vi "Persistent.vi"(7 "Field monitor ref":refnum<vi>, 8 "error in (no error)":errorcluster, 10 "Go to persistent mode?":bool, 11 "Power Supply in":refnum<class "Power Supply.lvclass">) -> (0 "error out":errorcluster, 3 "Power Supply out":refnum<class "Power Supply.lvclass">)   [LabVIEW 2009, in "Power Supply.lvclass"]
doc: "Persistent mode closes the switch and turns off the power supply. The superconducting electromagnet will then remain energized indefinitely.\n\nTo leave persistent mode, you must first ramp up the power supply to match the energized magnet, then open the switch. \n\nA current mismatch is dangerous! The magnet will forbid opening the switch unless the power supply matches the energized magnet."
uses:
  Power Supply.lvclass
  Global/Relative Sound Files.vi
panel:
  out "SHon?":bool caption="Switch Heater"
  out "persis?":bool caption="Persistent"
  out "title":string
  out "Field":dbl[unit]
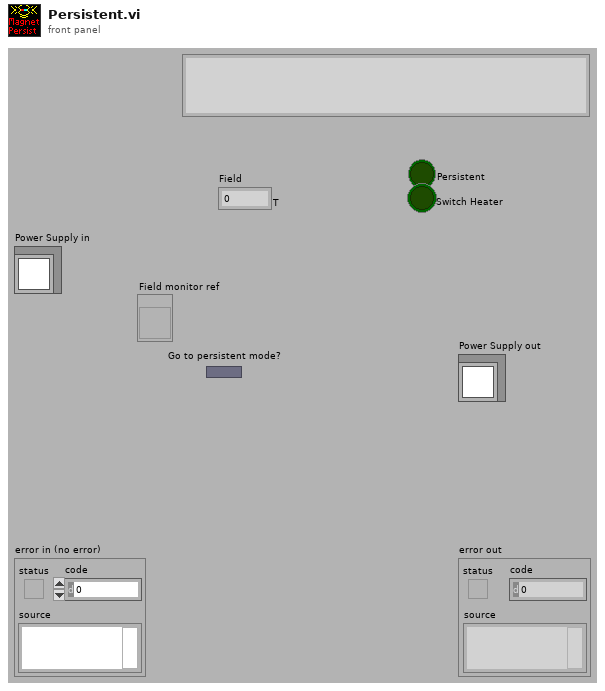
[diagram p1: front panel]
types:
  T1 = typedef "Power Supply.lvclass/Switch Heater Status.ctl" = enum16{"Off (at zero)", "On", "Off (at field)", "Other"}
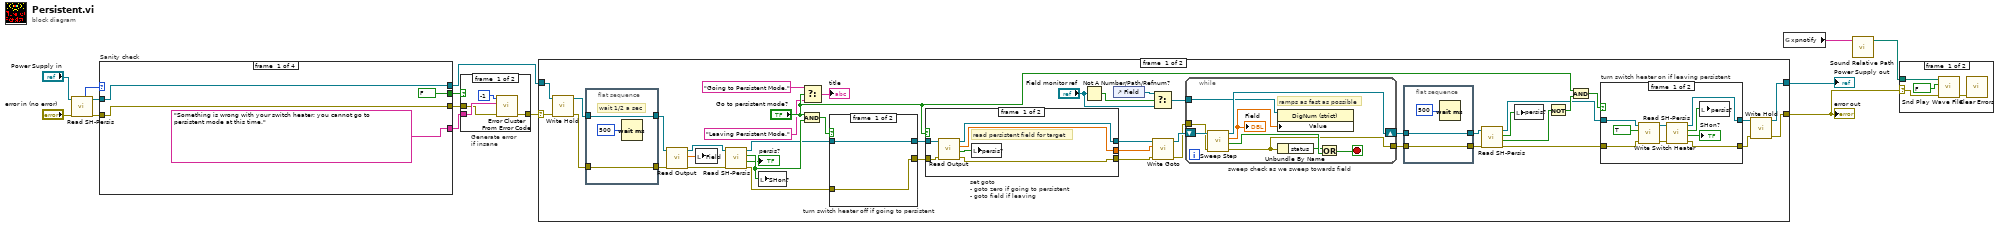
[diagram p0: block diagram]
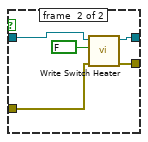
[diagram p2: hidden frame]
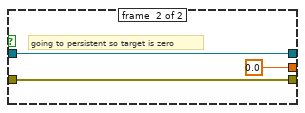
[diagram p3: hidden frame]
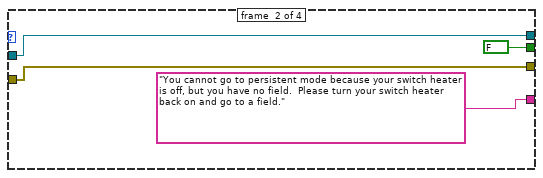
[diagram p7: hidden frame]
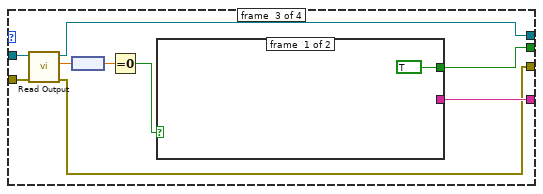
[diagram p8: hidden frame]
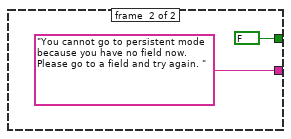
[diagram p9: hidden frame]
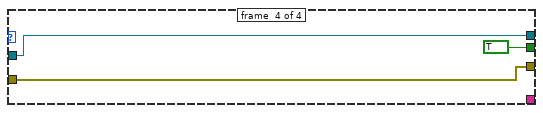
[diagram p10: hidden frame]
diagram:
  n1 = call-dynamic "Read SH-Persis.vi"("error in (no error)"="error in (no error)", "Power Supply in"="Power Supply in") -> ("error out"=w6:errorcluster, "Power Supply out"=w8:refnum<class "Power Supply.lvclass">, "SHstatus"=w11:T1)  [unwired: 4 in, 3 out]
  n2 = case "Sanity check" shown="\"Off (at field)\"" w11 {
    tunnel: [FALSE FALSE w31 TRUE] -> w10
    tunnel: ["Something is wrong with your switch heater; you cannot go to persistent mode at this time." "You cannot go to persistent mode because your switch heater is off, but you have no field.  Please turn your switch heater back on and go to a field." w28 _] -> w9
    tunnel: w8 -> [w16 w20 w27 w36]
    tunnel: [w16 w20 w26 w36] -> w12
    tunnel: [w15 w19 w25 w35] -> w7
    tunnel: w6 -> [w15 w19 w24 w35]
    frame #0 {
    }
    frame #1 {
    }
    frame #2 {
      n3 = call-dynamic "Read Output.vi"("error in (no error)"=w24, "Power Supply in"=w27) -> ("error out"=w25:errorcluster, "Field"=w30:dbl[unit], "Power Supply out"=w26:refnum<class "Power Supply.lvclass">)  [unwired: 6 in, 1 out]
      n4 = node(w30) -> (w23:dbl)
      n5 = Equal To 0?(x=w23) -> (x = 0?=w29:bool)
      n6 = case shown="False" w29 {
        tunnel: [TRUE FALSE] -> w31
        tunnel: [_ "You cannot go to persistent mode because you have no field now.  Please go to a field and try again. "] -> w28
        frame #0 {
        }
        frame #1 {
        }
      }
    }
    frame #3 {
    }
  }
  n7 = case "Generate error\nif insane" shown="True" w10 {
    tunnel: w9 -> [w40 _]
    tunnel: [w39 w42] -> w4
    tunnel: w7 -> [w38 w42]
    frame #0 {
      n8 = call <vilib>:"Error Cluster From Error Code.vi"("error in (no error)"=w38, "error message (\"\")"=w40, "error code (0)"=-1) -> ("error out"=w39:errorcluster)  [unwired: 6 in]
    }
    frame #1 {
    }
  }
  n9 = case shown="No Error" w4 {
    selector: w4 -> [w47 w129]
    tunnel: [w84 w128] -> w13
    tunnel: [w83 w129] -> w3
    tunnel: w12 -> [w52 w128]
    frame #0 {
      n10 = call-dynamic "Write Hold.vi"("error in (no error)"=w47, "Power Supply in"=w52) -> ("error out"=w48:errorcluster, "Power Supply out"=w51:refnum<class "Power Supply.lvclass">)  [unwired: 8 in]
      n11 = flat-sequence {
        tunnel: w51 -> [w88]
        tunnel: [w88] -> w50
        tunnel: [w87] -> w49
        tunnel: w48 -> [w87]
        frame #0 {
          # "wait 1/2 a sec"
          n12 = Wait (ms)(milliseconds to wait=500) -> ()  [unwired: 1 out]
        }
      }
      n13 = call-dynamic "Read Output.vi"("error in (no error)"=w49, "Power Supply in"=w50) -> ("error out"=w59:errorcluster, "Field"=w53:dbl[unit], "Power Supply out"=w60:refnum<class "Power Supply.lvclass">)  [unwired: 6 in, 1 out]
      n14 = local write "Field"(w53) -> ()
      n15 = call-dynamic "Read SH-Persis.vi"("error in (no error)"=w59, "Power Supply in"=w60) -> ("error out"=w57:errorcluster, "SHon?"=w62:bool, "pers?"=→"persis?":bool, "Power Supply out"=w58:refnum<class "Power Supply.lvclass">)  [unwired: 4 in, 2 out]
      n16 = local write "SHon?"(w62) -> ()
      n17 = And(x="Go to persistent mode?", y=w62) -> (x .and. y?=w63:bool)
      n18 = Select(t="Going to Persistent Mode.", s="Go to persistent mode?", f="Leaving Persistent Mode.") -> (s? t:f=→"title":string)
      n19 = case "turn switch heater off if going to persistent" shown="True" w63 {
        tunnel: [w90 w93] -> w66
        tunnel: w58 -> [w90 w94]
        tunnel: w57 -> [w89 w92]
        tunnel: [w89 w91] -> w65
        frame #0 {
        }
        frame #1 {
          n20 = call-dynamic "Write Switch Heater.vi"("error in (no error)"=w92, "Turn SH On?"=FALSE, "Power Supply in"=w94) -> ("error out"=w91:errorcluster, "Power Supply out"=w93:refnum<class "Power Supply.lvclass">)  [unwired: 7 in]
        }
      }
      n21 = case "set goto\n- goto zero if going to persistent\n- goto field if leaving" shown="True" "Go to persistent mode?" {
        tunnel: [w100 dbl[unit] 0.0 ("Field")] -> w68
        tunnel: [w99 w103] -> w67
        tunnel: w66 -> [w98 w103]
        tunnel: w65 -> [w97 w102]
        tunnel: [w96 w102] -> w64
        frame #0 {
          # "read persistent field for target"
          n22 = call-dynamic "Read Output.vi"("error in (no error)"=w97, "Power Supply in"=w98) -> ("error out"=w96:errorcluster, "persistent?"=w101:bool, "Field"=w100:dbl[unit], "Power Supply out"=w99:refnum<class "Power Supply.lvclass">)  [unwired: 6 in]
          n23 = local write "persis?"(w101) -> ()
        }
        frame #1 {
          # "going to persistent so target is zero"
        }
      }
      n24 = Not A Number/Path/Refnum?(number/path/refnum="Field monitor ref") -> (NaN/Path/Refnum?=w46:bool)
      n25 = control-ref of="Field"() -> (w45:refnum<vi>)
      n26 = Select(t=w45, s=w46, f="Field monitor ref") -> (s? t:f=w43:refnum<vi>)
      n27 = call-dynamic "Write Goto.vi"("error in (no error)"=w64, "Target"=w68, "Power Supply in"=w67) -> ("error out"=w69:errorcluster, "Power Supply out"=w70:refnum<class "Power Supply.lvclass">)  [unwired: 7 in]
      n28 = while "sweep check as we sweep towards field" {
        shift-right: [w112] -> w72
        shift-left: w70 -> [w113]
        tunnel: [w106] -> w71
        tunnel: w69 -> [w110]
        tunnel: w43 -> [w109]
        stop <- w107 stop-if-true
        # "ramps as fast as possible"
        n29 = call-dynamic "Sweep Step.vi"("error in (no error)"=w110, "Power Supply in"=w113) -> ("error out"=w106:errorcluster, "Done?"=w111:bool, "field"=w108:dbl[unit], "Power Supply out"=w112:refnum<class "Power Supply.lvclass">)  [unwired: 5 in, 1 out]
        "Field" <- w108
        n30 = property on="Property Node" class="DigNum (strict)"(reference=w109, "Value"=w108) -> ()  [unwired: 1 in, 2 out]
        n31 = Unbundle By Name(w106) -> ("status"=w105:bool)
        n32 = Or(x=w105, y=w111) -> (x .or. y?=w107:bool)
      }
      n33 = flat-sequence {
        tunnel: w72 -> [w115]
        tunnel: [w115] -> w76
        tunnel: w71 -> [w114]
        tunnel: [w114] -> w75
        frame #0 {
          n34 = Wait (ms)(milliseconds to wait=500) -> ()  [unwired: 1 out]
        }
      }
      n35 = call-dynamic "Read SH-Persis.vi"("error in (no error)"=w75, "Power Supply in"=w76) -> ("error out"=w74:errorcluster, "SHon?"=w78:bool, "pers?"=w77:bool, "Power Supply out"=w73:refnum<class "Power Supply.lvclass">)  [unwired: 4 in, 2 out]
      n36 = local write "persis?"(w77) -> ()
      n37 = Not(x=w78) -> (.not. x?=w79:bool)
      n38 = And(x="Go to persistent mode?", y=w79) -> (x .and. y?=w80:bool)
      n39 = case "turn switch heater on if leaving persistent" shown="False" w80 {
        tunnel: [w121 w126] -> w81
        tunnel: w74 -> [w124 w126]
        tunnel: w73 -> [w125 w127]
        tunnel: [w117 w127] -> w82
        frame #0 {
          n40 = call-dynamic "Write Switch Heater.vi"("error in (no error)"=w124, "Turn SH On?"=TRUE, "Power Supply in"=w125) -> ("error out"=w122:errorcluster, "Power Supply out"=w118:refnum<class "Power Supply.lvclass">)  [unwired: 7 in]
          n41 = call-dynamic "Read SH-Persis.vi"("error in (no error)"=w122, "Power Supply in"=w118) -> ("error out"=w121:errorcluster, "SHon?"=→"SHon?":bool, "pers?"=w119:bool, "Power Supply out"=w117:refnum<class "Power Supply.lvclass">)  [unwired: 4 in, 2 out]
          n42 = local write "persis?"(w119) -> ()
        }
        frame #1 {
        }
      }
      n43 = call-dynamic "Write Hold.vi"("error in (no error)"=w81, "Power Supply in"=w82) -> ("error out"=w83:errorcluster, "Power Supply out"=w84:refnum<class "Power Supply.lvclass">)  [unwired: 8 in]
    }
    frame #1 {
    }
  }
  "Power Supply out" <- w13
  "error out" <- w3
  n44 = global read "Relative Sound Files.vi" "xpnotify"() -> (w2:string)
  n45 = call "Sound Relative Path.vi"("Sound"=w2) -> ("Relative Path"=w1:path)  [unwired: 10 in]
  n46 = case shown="No Error" w3 {
    selector: w3 -> [w130 _]
    tunnel: w1 -> [w133 _]
    frame #0 {
      n47 = call <vilib>:"Snd Play Wave File.vi"("error in (no error)"=w130, "wait until finish (T)"=FALSE, "wave file path"=w133) -> ("error out"=w131:errorcluster)  [unwired: 8 out]
      n48 = call <vilib>:"Clear Errors.vi"("error in (no error)"=w131) -> ()  [unwired: 6 in, 1 out]
    }
    frame #1 {
    }
  }
